vi "DSF.Engine.Pointer.VS Channels.New.vi"(8 "error in (no error)":errorcluster, 10 "channel count":u64, 11 "Data Reference":T1 format="%.0x") -> (0 "error out":errorcluster, 3 "VS Channels Pointer out":refnum<class "DSF.Engine.Pointer.VS Channels.lvclass">)   [LabVIEW 2016, in "DSF.Engine.lvlib" / "DSF.Engine.Pointer.VS Channels.lvclass"]
uses:
  DSF.Engine.Pointer.VS Channels.lvclass
  C:/Program Files (x86)/National Instruments/LabVIEW 2016/vi.lib/National Instruments/Memory Manager/Classes/Pointer/Memory.Pointer.lvclass
  <vilib>/NI Veristand/Custom Device API/Data Reference.ctl
  Shared/Typedefs/DSF.Shared.Typedefs.Data Type.ctl
  <vilib>/National Instruments/Memory Manager/Classes/Pointer/Memory.Pointer.lvclass/Memory.Pointer.ctl
  Shared/VIs/DSF.Shared.Data Type.Sizeof.vi
  <vilib>/National Instruments/Memory Manager/Classes/Pointer/Memory.Pointer.Set Size.vi
  <vilib>/National Instruments/Memory Manager/Classes/Pointer/Memory.Pointer.Set Address.vi
  <vilib>/National Instruments/Memory Manager/Classes/Pointer/Memory.Pointer.Parameter Check.Null Pointer.vi
  <vilib>/National Instruments/Memory Manager/Classes/Pointer/Memory.Pointer.Set Allocated.vi
  <vilib>/National Instruments/Memory Manager/Classes/Pointer/Memory.Pointer.Errors.vi
  <vilib>/National Instruments/Memory Manager/Classes/Pointer/Memory.Pointer.Errors.Null Pointer.vi
  <vilib>/National Instruments/Memory Manager/Classes/Pointer/Memory.Pointer.Get Address.vi
  <vilib>/National Instruments/Memory Manager/Classes/Pointer/Memory.Pointer.Errors.Create Error.vi
  <vilib>/National Instruments/Memory Manager/Constants/Memory.Constants.vi
  <vilib>/National Instruments/Memory Manager/Constants/Memory.Constants.Library Name.vi
  <vilib>/National Instruments/Memory Manager/Classes/Pointer/Memory.Pointer.Errors.Get Info.vi
  <vilib>/National Instruments/Memory Manager/Submodules/SEH/Source/VIs/Static Error Handling.Source Buffer.Write.String.vi
  <vilib>/National Instruments/Memory Manager/Submodules/SEH/Source/VIs/Static Error Handling.Parameters.VI Source.Set.vi
  <vilib>/National Instruments/Memory Manager/Submodules/SEH/Source/VIs/Static Error Handling.Parameters.Code.Set.vi
  <vilib>/National Instruments/Memory Manager/Submodules/SEH/Source/VIs/Static Error Handling.Parameters.Status.Set.vi
  <vilib>/National Instruments/Memory Manager/Submodules/SEH/Source/VIs/Static Error Handling.Error Cluster Constant.vi
  <vilib>/National Instruments/Memory Manager/Submodules/SEH/Source/VIs/Static Error Handling.Error Cluster Constant (512B).vi
  <vilib>/NI Veristand/Custom Device API/Global Data Refs.vi
  DSF.Shared.lvlib
  <vilib>/National Instruments/Memory Manager/Classes/Pointer/Memory.Pointer.lvclass
  <vilib>/NI Veristand/Custom Device API/Custom Device API.lvlib
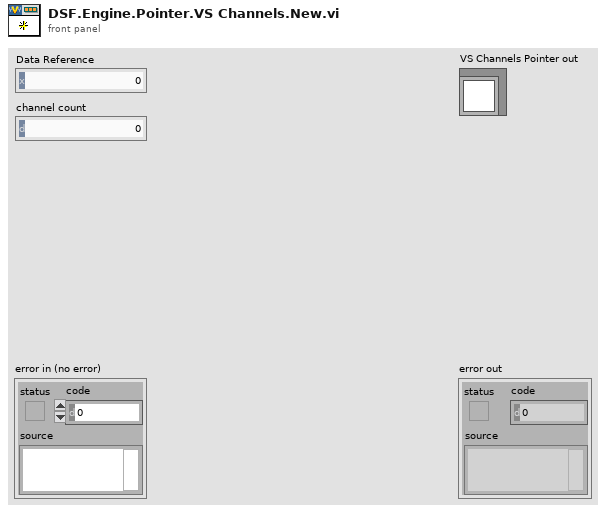
[diagram p1: front panel]
types:
  T1 = typedef "Custom Device API.lvlib/Data Reference.ctl" = i32
  T2 = typedef "DSF.Shared.lvlib/DSF.Shared.Typedefs.Data Type.ctl" = enum8{"Bool", "SGL", "DBL", "I8", "I16", "I32", "I64", "U8", "U16", "U32", "U64"}
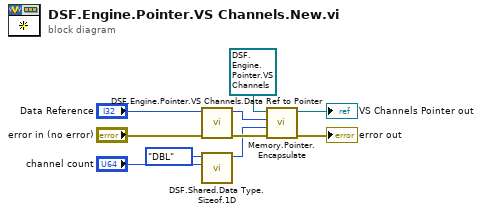
[diagram p0: block diagram]
diagram:
  n1 = call "DSF.Engine.Pointer.VS Channels.Data Ref to Pointer.vi"("error in (no error)"="error in (no error)", "Data Reference"="Data Reference") -> ("error out"=w6:errorcluster, "Channel Pointer"=w4:u64)  [unwired: 8 in]
  n2 = call "DSF.Shared.Data Type.Sizeof.1D.vi"("count"="channel count", "data type"=DSF.Shared.Typedefs.Data_Type."DBL") -> ("size in bytes"=w3:u64)  [unwired: 9 in]
  n3 = call <vilib>:"Memory.Pointer.Encapsulate.vi"("error in (no error)"=w6, "size"=w3, "address"=w4, "Pointer type"=refnum<class "DSF.Engine.Pointer.VS Channels.lvclass"> refnum ("VS Channels Pointer out")) -> ("error out"=→"error out":errorcluster, "Pointer out"=→"VS Channels Pointer out":refnum<class "DSF.Engine.Pointer.VS Channels.lvclass">)  [unwired: 6 in]
